vi "WriteVerify Mfg Test Timestamp.vi"(8 "error in":errorcluster) -> (0 "error out":errorcluster)   [LabVIEW 2015]
panel:
  out "Delta Time":dbl
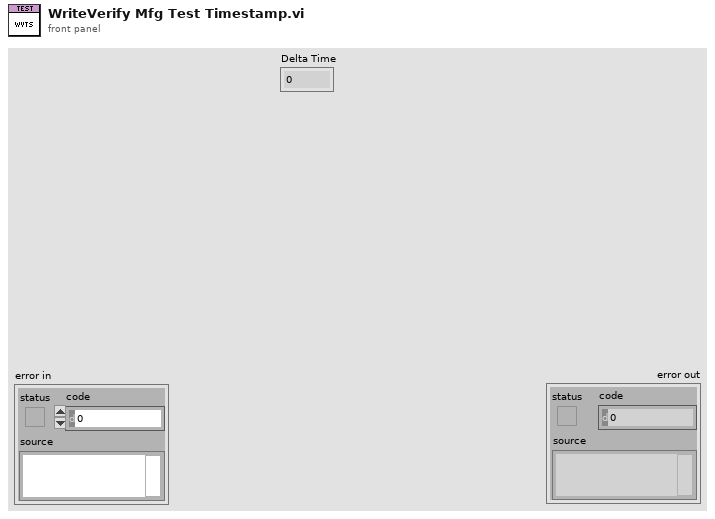
[diagram p1: front panel]
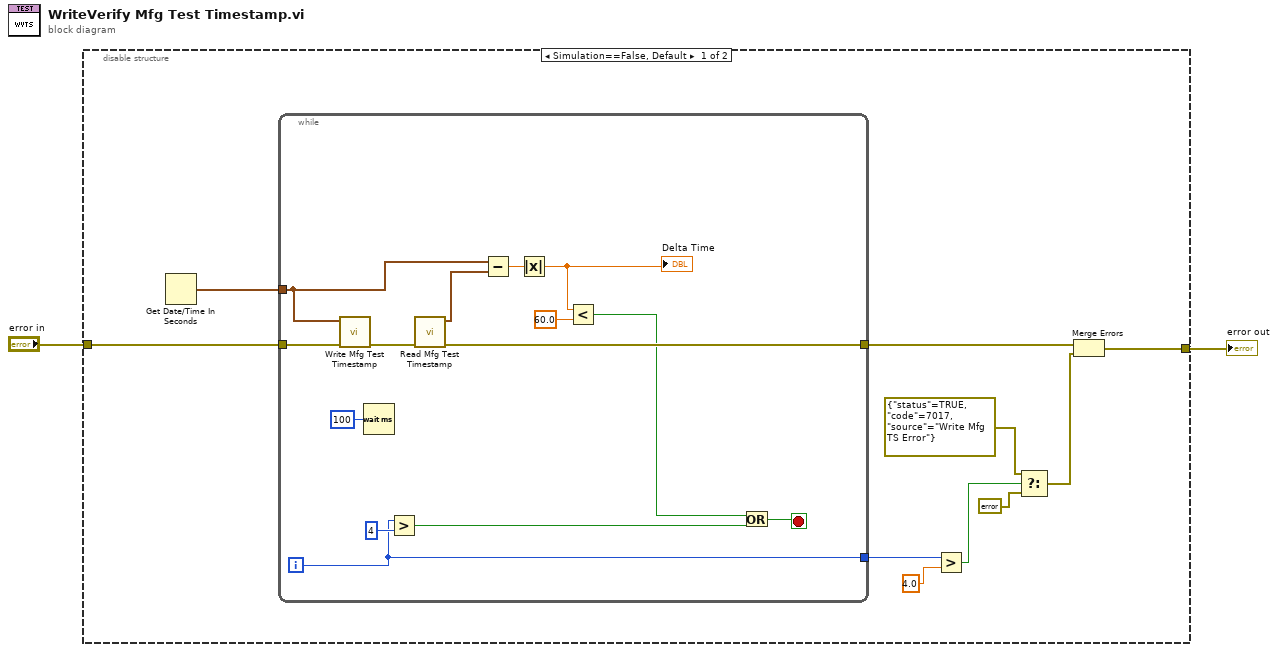
[diagram p0: block diagram]
diagram:
  n1 = disable-structure shown="Simulation==False, Default" {
    disable-tunnel: "error in" -> [w12 w27]
    disable-tunnel: [w4 w27] -> w1
    frame condition #0 (active) {
      n2 = Get Date/Time In Seconds() -> (seconds since 1Jan1904=w3:timestamp)
      n3 = while {
        tunnel: w12 -> [w26]
        tunnel: [w15] -> w5
        tunnel: [w21] -> w10
        tunnel: w3 -> [w13]
        i -> [w21]
        stop <- w23 stop-if-true
        n4 = call "Write Mfg Test Timestamp.vi"("error in"=w26, "Time Stamp"=w13) -> ("error out"=w20:errorcluster)  [unwired: 9 in]
        n5 = Wait (ms)(milliseconds to wait=u32 100) -> ()  [unwired: 1 out]
        n6 = Greater?(x=w21, y=4) -> (0:w24:bool)
        n7 = call "Read Mfg Test Timestamp.vi"("error in"=w20) -> ("error out"=w15:errorcluster, "time stamp"=w19:timestamp)  [unwired: 9 in]
        n8 = Subtract(x=w13, y=w19) -> (x-y=w18:dbl)
        n9 = Absolute Value(x=w18) -> (abs(x)=w17:dbl)
        "Delta Time" <- w17
        n10 = Less?(x=w17, y=60.0) -> (x < y?=w14:bool)
        n11 = Or(x=w14, y=w24) -> (x .or. y?=w23:bool)
      }
      n12 = Greater?(x=w10, y=4.0) -> (0:w9:bool)
      n13 = Select(t=errorcluster {"status"=TRUE, "code"=7017, "source"="Write Mfg TS Error"} ("f"), s=w9, f=errorcluster {"status"=FALSE, "code"=0, "source"=""}) -> (s? t:f=w6:errorcluster)
      n14 = Merge Errors(w5, w6) -> (w4:errorcluster)
    }
    frame condition #1 {
    }
  }
  "error out" <- w1
